vi "Create Message.vi"   [LabVIEW 2015, in "TLB` Template.lvlib" / "AMC.lvlib"]
doc: "Creates an AMC message, which can be passed to Send Message.vi.TLB Prime - Application Template 1.3.0.24\nNorm Kirchner, NI Systems Engineering - NI\nCopyright (c) 2014, NI"
uses:
  AMC.lvlib
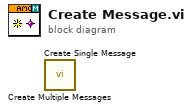
[diagram p0: block diagram]
diagram:
  n1 = call "Create Multiple Messages.vi"() -> ()  [unwired: 14 in, 2 out]
  n2 = call "Create Single Message.vi"() -> ()  [unwired: 14 in, 2 out]
